vi "Wrap.vi"(8 "Error In":errorcluster, 10 "Arrays":u8[](array[numeric]), 11 "ByteBuffer In":refnum<class "ByteBuffer.lvclass">) -> (0 "Error Out":errorcluster, 3 "ByteBuffer Out":refnum<class "ByteBuffer.lvclass">)   [LabVIEW 2015, in "ByteBuffer.lvclass"]
doc: "Wraps a byte array into a buffer.\nThe new buffer will be backed by the given byte array; that is, modifications to the buffer will cause the array to be modified and vice versa. The new buffer's capacity and limit will be array.length, its position will be zero, and its mark will be undefined. Its backing array will be the given array, and its array offset will be zero.\n\nParameters:\n+ Array - The array that will back this buffer.\n\nReturns:\nThe new byte buffer."
uses:
  ByteBuffer.lvclass
  ByteBuffer.lvclass/ByteBuffer.ctl
  <vilib>/Utility/error.llb/Error Cluster From Error Code.vi
  <vilib>/ErrorRing/Error Ring.xnode
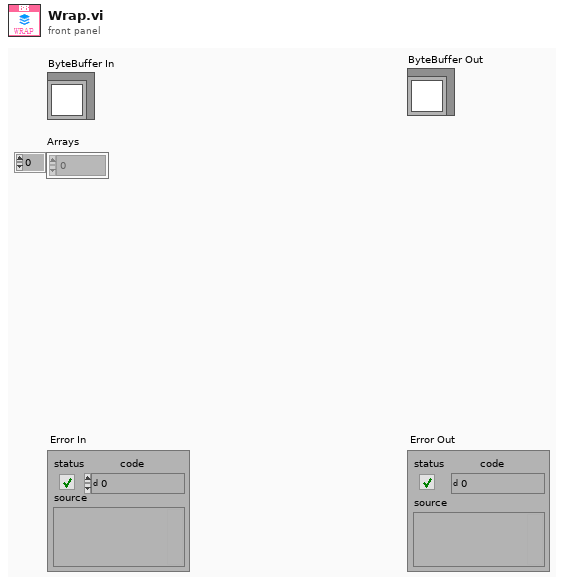
[diagram p1: front panel]
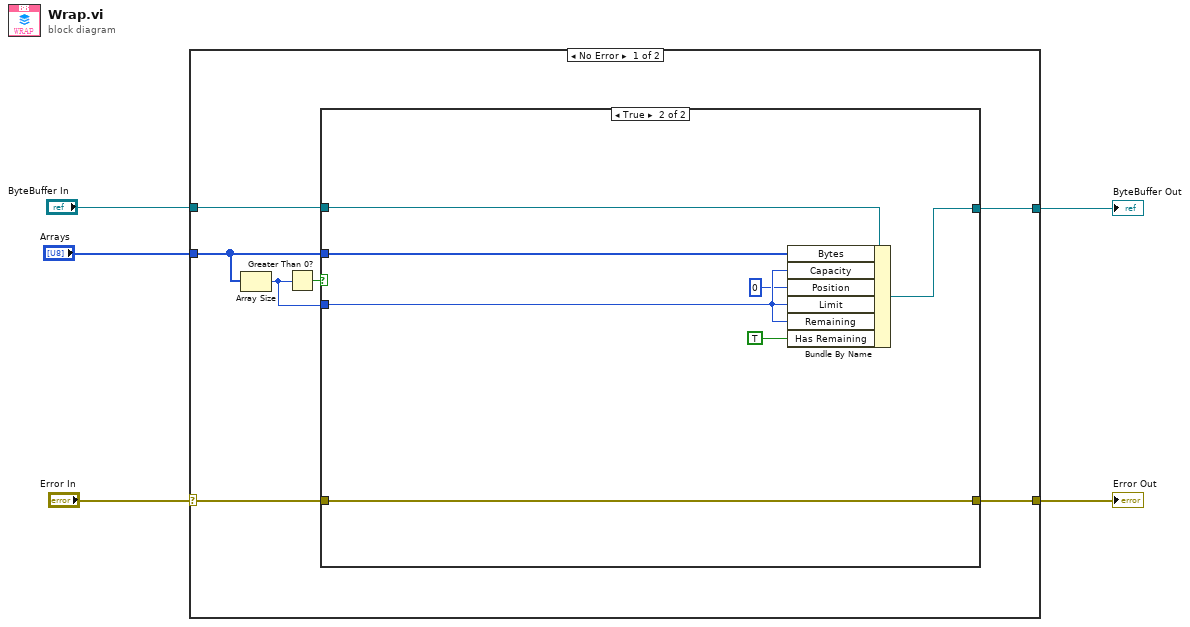
[diagram p0: block diagram]
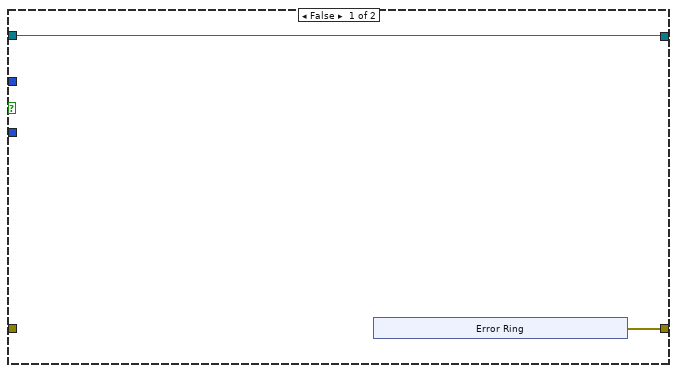
[diagram p2: hidden frame]
diagram:
  n1 = case shown="No Error" "Error In" {
    selector: "Error In" -> [w8 w28]
    tunnel: "ByteBuffer In" -> [w12 w27]
    tunnel: [w11 w27] -> w4
    tunnel: "Arrays" -> [w10 _]
    tunnel: [w7 w28] -> w1
    frame No Error {
      n2 = Array Size(array=w10) -> (size(s)=w6:i32)
      n3 = Greater Than 0?(x=w6) -> (x > 0?=w9:bool)
      n4 = case shown="True" w9 {
        tunnel: w12 -> [w14 w26]
        tunnel: [w14 w25] -> w11
        tunnel: w10 -> [_ w24]
        tunnel: w8 -> [_ w23]
        tunnel: [w13 w23] -> w7
        tunnel: w6 -> [_ w22]
        frame False {
          n5 = xnode "Error Ring"() -> ("error out"=w13:errorcluster)
        }
        frame True {
          n6 = Bundle By Name(cluster=w26, "Bytes"=w24, "Capacity"=w22, "Position"=u32 0, "Limit"=w22, "Remaining"=w22, "Has Remaining"=TRUE) -> (w25:refnum<class "ByteBuffer.lvclass">)
        }
      }
    }
    frame Error {
    }
  }
  "ByteBuffer Out" <- w4
  "Error Out" <- w1
